vi "DrawPiePlot.vi"(0 "reference in":refnum<class "LcWebView.lvclass">, 1 "PiePlot.PlotLabels":string[](array[string]), 2 "PiePlot.Dataset":dbl[][](array[numeric]), 3 "PiePlot.DatasetLabels":string[](array[string]), 5 "Error In":errorcluster, 6 "GenericPlotOptions":T1, 7 "PiePlot.PlotColours":u32[](array[numeric]), 8 "PiePlotOptions":T3) -> (14 "reference out":refnum<class "LcWebView.lvclass">, 19 "Error Out":errorcluster)   [LabVIEW 2018, in "LcWebView.lvclass"]
uses:
  LcWebView.lvclass
  ctrls/PiePlotOption.ctl
  ctrls/GenericPlotOption.ctl
  ctrls/LegendPosition.ctl
  ctrls/GenericPlotOption_NoEnumPrivate.ctl
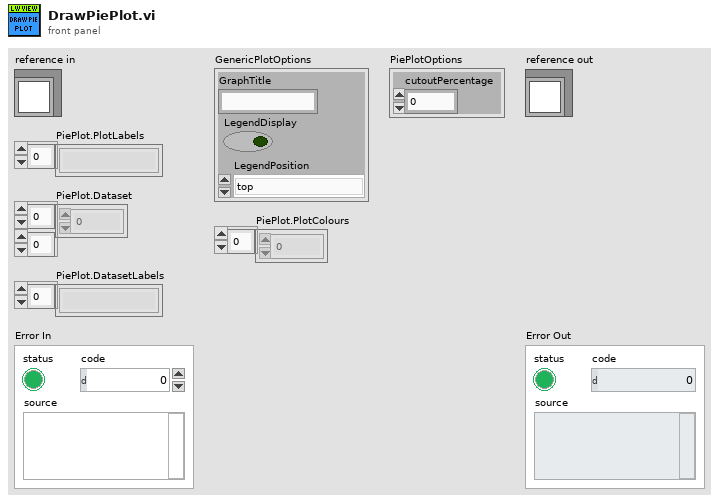
[diagram p1: front panel]
types:
  T1 = typedef "LcWebView.lvclass/GenericPlotOption.ctl" = cluster{"GraphTitle":string, "LegendDisplay":bool, "LegendPosition":T2}
  T2 = typedef "LcWebView.lvclass/LegendPosition.ctl" = enum16{"top", "right", "left", "bottom"}
  T3 = typedef "LcWebView.lvclass/PiePlotOption.ctl" = cluster{"cutoutPercentage":i32}
  T4 = typedef "LcWebView.lvclass/GenericPlotOption_NoEnumPrivate.ctl" = cluster{"GraphTitle":string, "LegendDisplay":bool, "LegendPosition":string}
  T5 = cluster{"action":string, "PlotData":string, "GenericPlotOptions":T4, "PiePlotOptions":T3}
  T6 = cluster{"GraphTitle":string, "LegendDisplay":bool, "LegendPosition":string}
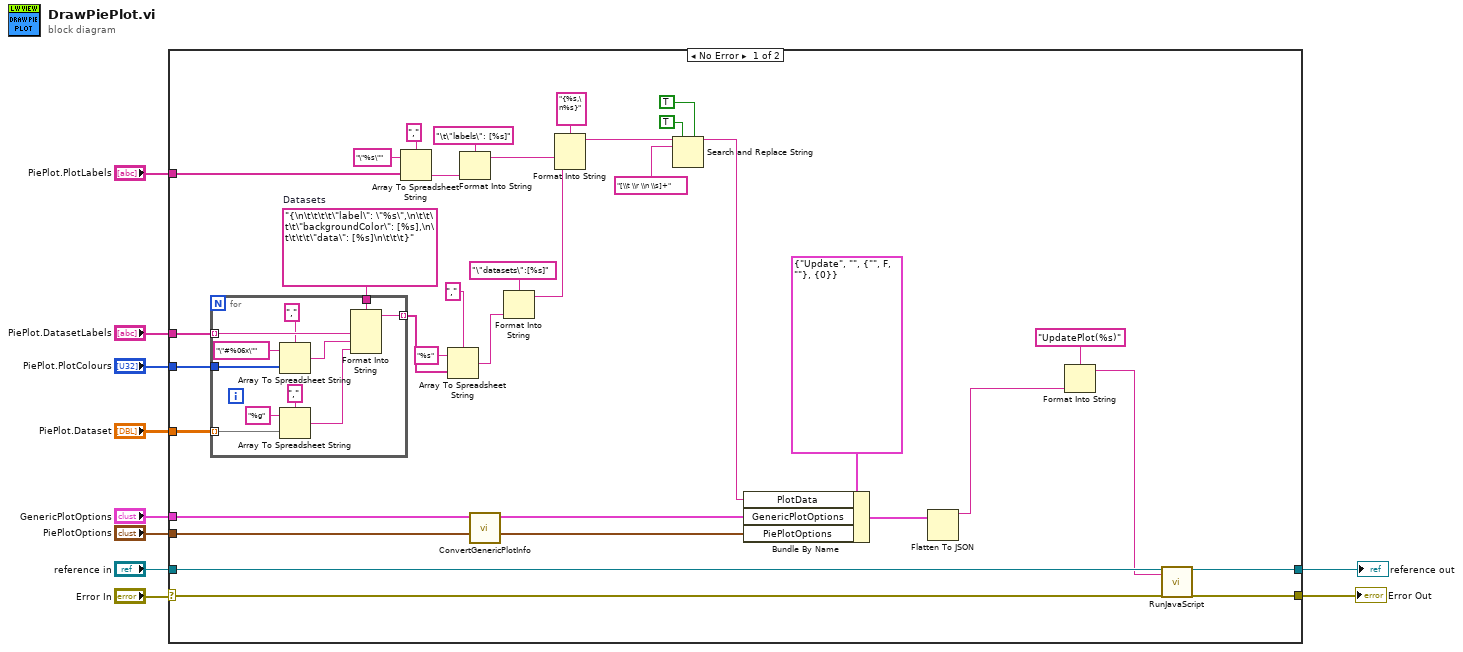
[diagram p0: block diagram]
diagram:
  n1 = case shown="No Error" "Error In" {
    selector: "Error In" -> [w23 w57]
    tunnel: [w17 w57] -> w4
    tunnel: [w18 w56] -> w1
    tunnel: "reference in" -> [w22 w56]
    tunnel: "PiePlot.Dataset" -> [w35 _]
    tunnel: "PiePlot.PlotColours" -> [w34 _]
    tunnel: "PiePlot.DatasetLabels" -> [w33 _]
    tunnel: "PiePlot.PlotLabels" -> [w32 _]
    tunnel: "GenericPlotOptions" -> [w26 _]
    tunnel: "PiePlotOptions" -> [w24 _]
    frame No Error {
      w36 = "{\n\t\t\t\t\"label\": \"%s\",\n\t\t\t\t\"backgroundColor\": [%s],\n\t\t\t\t\"data\": [%s]\n\t\t\t}"  # Datasets
      n2 = for {
        tunnel: w35 -> [w53] mode=indexing
        tunnel: w34 -> [w46]
        tunnel: w33 -> [w52] mode=indexing
        tunnel: [w50] -> w15 mode=indexing
        tunnel: w36 -> [w49]
        n3 = Array To Spreadsheet String(delimiter (Tab)=",", array=w46, 3:"\"#%06x\"" ("format string")) -> (spreadsheet string=w45:string)
        n4 = Array To Spreadsheet String(delimiter (Tab)=",", array=w53, 3:"%g" ("format string")) -> (spreadsheet string=w51:string)
        n5 = Format Into String(format string=w49, w52, w45, w51) -> (resulting string=w50:string)  [unwired: 2 in, 1 out]
      }
      n6 = Array To Spreadsheet String(delimiter (Tab)=",", array=w32, 3:"\"%s\"" ("format string")) -> (spreadsheet string=w40:string)
      n7 = Array To Spreadsheet String(delimiter (Tab)="," ("separator"), array=w15, 3:"%s" ("format string")) -> (spreadsheet string=w12:string)
      n8 = Format Into String(format string="\t\"labels\": [%s]", w40) -> (resulting string=w43:string)  [unwired: 2 in, 1 out]
      n9 = call "ConvertGenericPlotInfo.vi"("GenericPlotOptions in"=w26) -> ("GenericPlotOptionsOut(NoEnum)"=w11:T6)  [unwired: 10 in]
      n10 = Format Into String(format string="\"datasets\":[%s]", w12) -> (resulting string=w38:string)  [unwired: 2 in, 1 out]
      n11 = Format Into String(format string="{%s,\n%s}", w43, w38) -> (resulting string=w25:string)  [unwired: 2 in, 1 out]
      n12 = Search and Replace String(replace all?=TRUE ("replace all? (F)"), multiline?=TRUE ("multiline? (F)"), input string=w25, search string="[\\t \\r \\n \\s]+") -> (result string=w31:string)  [unwired: 4 in, 3 out]
      n13 = Bundle By Name(cluster=T5 {"action"="Update", "PlotData"="", "GenericPlotOptions"={"GraphTitle"="", "LegendDisplay"=FALSE, "LegendPosition"=""}, "PiePlotOptions"={"cutoutPercentage"=0}}, "PlotData"=w31, "GenericPlotOptions"=w11, "PiePlotOptions"=w24) -> (w21:T5)
      n14 = Flatten To JSON(anything=w21) -> (JSON string=w19:string)  [unwired: 2 in, 1 out]
      n15 = Format Into String(format string="UpdatePlot(%s)", w19) -> (resulting string=w16:string)  [unwired: 2 in, 1 out]
      n16 = call-dynamic "RunJavaScript.vi"("reference in"=w22, "Java Script Function"=w16, "Error In"=w23) -> ("reference out"=w18:refnum<class "LcWebView.lvclass">, "Error Out"=w17:errorcluster)  [unwired: 13 in, 2 out]
    }
    frame Error {
    }
  }
  "Error Out" <- w4
  "reference out" <- w1
